vi "UpdateIntegration.vi"(2 "error in (no error)":errorcluster, 4 "EpiWrapper in":refnum<class "EpiWrapper.lvclass">) -> (0 "error out":errorcluster, 1 "EpiWrapper out":refnum<class "EpiWrapper.lvclass">)   [LabVIEW 2012, in "EpiWrapper.lvclass"]
uses:
  EpiWrapper.lvclass
  EpiWrapper.lvclass/EpiWrapper.ctl
  Instruments.lvclass
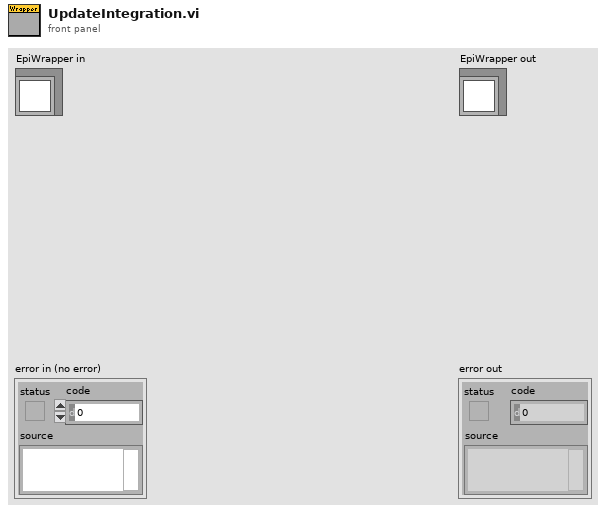
[diagram p1: front panel]
types:
  T1 = typedef "Config.ctl" = cluster{"IntTime":i32, "Samples":i32, "PowerMin":dbl, "KneeMin":dbl, "KneeMax":dbl, "Background Wl":dbl, "Settle Delay,ms":u32, "StationId":sgl}
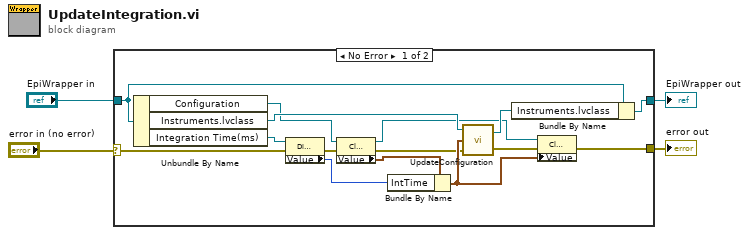
[diagram p0: block diagram]
diagram:
  n1 = case shown="No Error" "error in (no error)" {
    selector: "error in (no error)" -> [w13 w21]
    tunnel: [w6 w21] -> w3
    tunnel: [w16 w20] -> w1
    tunnel: "EpiWrapper in" -> [w18 w20]
    frame No Error {
      n2 = Unbundle By Name(w18) -> ("Configuration"=w9:refnum<vi>, "Instruments.lvclass"=w19:refnum<class "Instruments.lvclass">, "Integration Time(ms)"=w15:refnum<vi>)
      n3 = property class="DigNum (strict)"(reference=w15, error in=w13) -> (error out=w12:errorcluster, "Value"=w14:i32)  [unwired: 1 out]
      n4 = property class="Clust (strict)"(reference=w9, error in=w12) -> (reference out=w7:refnum<vi>, error out=w5:errorcluster, "Value"=w11:T1)
      n5 = Bundle By Name(cluster=w11, "IntTime"=w14) -> (w10:T1)
      n6 = call-dynamic "UpdateConfiguration.vi"("error in (no error)"=w5, "INSTR_PARAM.Config"=w10, "Instruments in"=w19) -> ("error out"=w8:errorcluster, "Instruments out"=w17:refnum<class "Instruments.lvclass">)
      n7 = Bundle By Name(cluster=w18, "Instruments.lvclass"=w17) -> (w16:refnum<class "EpiWrapper.lvclass">)
      n8 = property class="Clust (strict)"(reference=w7, error in=w8, "Value"=w10) -> (error out=w6:errorcluster)  [unwired: 1 out]
    }
    frame Error {
    }
  }
  "error out" <- w3
  "EpiWrapper out" <- w1
